vi "Do.vi"(8 "error in":errorcluster, 10 "Actor in":refnum<class "Actor.lvclass">, 11 "Update TEC PID":refnum<class "Update TEC PID.lvclass">) -> (0 "error out":errorcluster, 2 "Actor out":refnum<class "Actor.lvclass">)   [LabVIEW 2014, in "TE Cooler.lvlib" / "Update TEC PID.lvclass"]
doc: "(<B>Filename</B>: Actor Framework.lvlib:Message.lvclass:Do.vi)\n\nDefines what a message does when it is received by an actor. Generally, a message instructs an actor to invoke one of its methods. By default, this method does nothing. A child class must override it to define behavior. Create a child class by using the Actor Framework Message Maker dialog box."
uses:
  Update TEC PID.lvclass
  <vilib>/ActorFramework/Actor/Actor.lvclass
  Update TEC PID.lvclass/Update TEC PID.ctl
  reusable/DAQ Device/Device/Device.lvclass
  reusable/DAQ Device/Device/Device.lvclass/Device.ctl
  SuperActor/Ex Nested.lvclass/Ex Nested.ctl
  Devices/TE Cooler/TE Cooler.lvclass
  reusable/DAQ Device/Device/Read Configurable Device.vi
  SuperActor/Read ID.vi
  SuperActor/Read Log Session.vi
  SuperActor/Read CVT Session.vi
  <userlib>/_Session Fwk/Session - Root.lvclass
  Devices/Configurable Device/Configurable Device.lvclass
  reusable/Session APIs/CVT/CVT.lvclass
  reusable/Session APIs/Session Log/System Log.lvclass
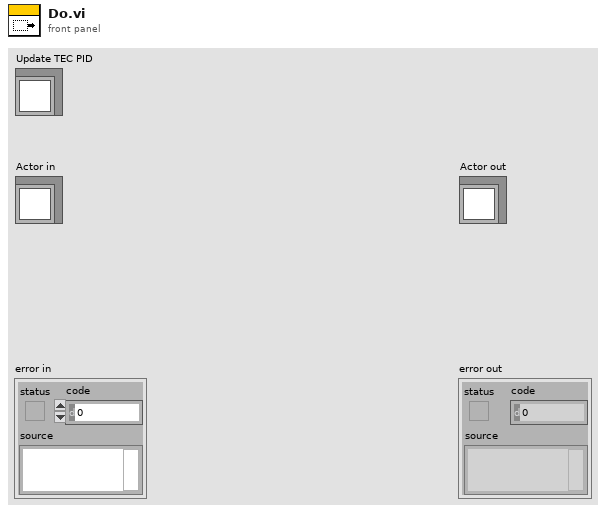
[diagram p1: front panel]
types:
  T1 = typedef "Session - Root.lvclass/Session Handle.ctl" = refnum<data-value>
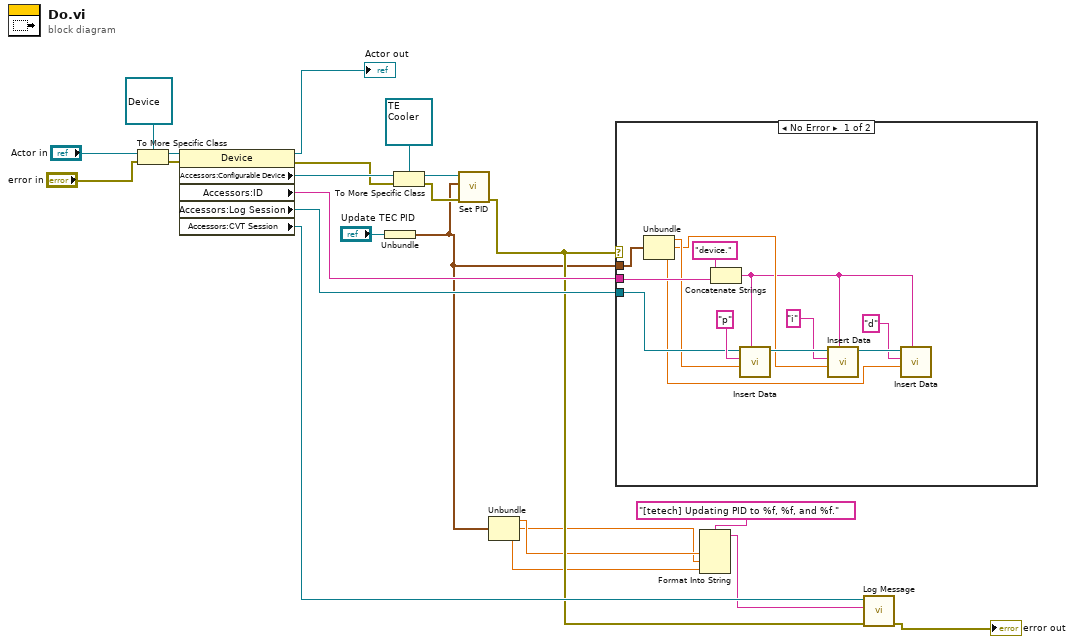
[diagram p0: block diagram]
diagram:
  n1 = To More Specific Class(target class=refnum<class "Device.lvclass"> refnum ("DAQ Device.lvlib:Device"), reference="Actor in", error in="error in") -> (specific class reference=w21:refnum<class "Device.lvclass">, error out=w14:errorcluster)
  n2 = property class="Device"(reference=w21, error in=w14) -> (reference out=→"Actor out":refnum<class "Device.lvclass">, error out=w18:errorcluster, "Accessors:Configurable Device"=w20:refnum<class "Configurable Device.lvclass">, "Accessors:ID"=w11:string, "Accessors:Log Session"=w12:T1, "Accessors:CVT Session"=w10:T1)
  n3 = Unbundle("Update TEC PID") -> (w7:cluster{"P":dbl, "I":dbl, "D":dbl})
  n4 = To More Specific Class(target class=refnum<class "TE Cooler.lvclass"> refnum ("TE Cooler.lvlib:TE Tech"), reference=w20, error in=w18) -> (specific class reference=w17:refnum<class "TE Cooler.lvclass">, error out=w16:errorcluster)
  n5 = call "Set PID.vi"("error in"=w16, "PID Params"=w7, "TE Cooler in"=w17) -> ("error out"=w9:errorcluster)  [unwired: 7 in, 1 out]
  n6 = Unbundle(w7) -> ("P"=w6:dbl, "I"=w5:dbl, "D"=w4:dbl)
  n7 = case shown="No Error" w9 {
    tunnel: w12 -> [w33 _]
    tunnel: w11 -> [w34 _]
    tunnel: w7 -> [w32 _]
    frame No Error {
      n8 = Unbundle(w32) -> ("P"=w31:dbl, "I"=w28:dbl, "D"=w24:dbl)
      n9 = Concatenate Strings("device." ("string"), w34) -> (w26:string)
      n10 = call "Insert Data.vi"("Group"=w26, "Data"=w31, "tag"="p", "CVT Session In"=w33) -> ("CVT Session Out"=w30:T1)  [unwired: 6 in, 1 out]
      n11 = call "Insert Data.vi"("Group"=w26, "Data"=w28, "tag"="i", "CVT Session In"=w30) -> ("CVT Session Out"=w27:T1)  [unwired: 6 in, 1 out]
      n12 = call "Insert Data.vi"("Group"=w26, "Data"=w24, "tag"="d", "CVT Session In"=w27) -> ()  [unwired: 6 in, 2 out]
    }
    frame Error {
    }
  }
  n13 = Format Into String(format string="[tetech] Updating PID to %f, %f, and %f.", w6, w5, w4) -> (resulting string=w3:string)  [unwired: 2 in, 1 out]
  n14 = call "Log Message.vi"("error in"=w9, "MSG In"=w3, "session in"=w10) -> ("error out"=→"error out":errorcluster)  [unwired: 7 in, 1 out]
